vi "updateItem.vi"(0 "reference in":refnum<class "Items Controller.lvclass">, 5 "dataIN":string[](array[string]), 7 "storageIN":string[][](array[string]), 9 "IN/OUT":bool, 11 "error in (no error)":errorcluster) -> (4 "reference out":refnum<class "Items Controller.lvclass">, 6 "found?":bool, 10 "storageOUT":string[][](array[string]), 15 "error out":errorcluster)   [LabVIEW 2014, in "Items Controller.lvclass"]
uses:
  Items Controller.lvclass
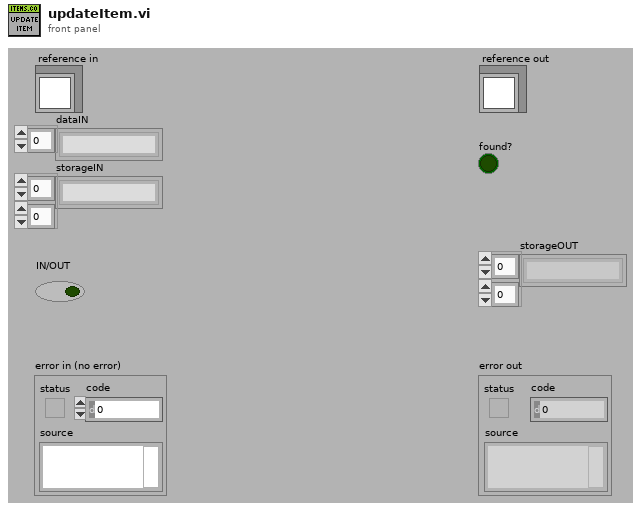
[diagram p1: front panel]
types:
  T1 = typedef "Items Controller.lvclass/ObjectAttributesRef.ctl" = refnum<data-value>
  T2 = typedef "Items Controller.lvclass/ObjectAttributes.ctl" = cluster{"MyAttribute":dbl, "data":string[][][], "file_controller_ref":refnum<class "File Controller.lvclass">, "checkIN_ref":refnum<class "checkIN.lvclass">, "checkOUT_ref":refnum<class "checkOUT.lvclass">, "item_ref":refnum<class "item.lvclass">}
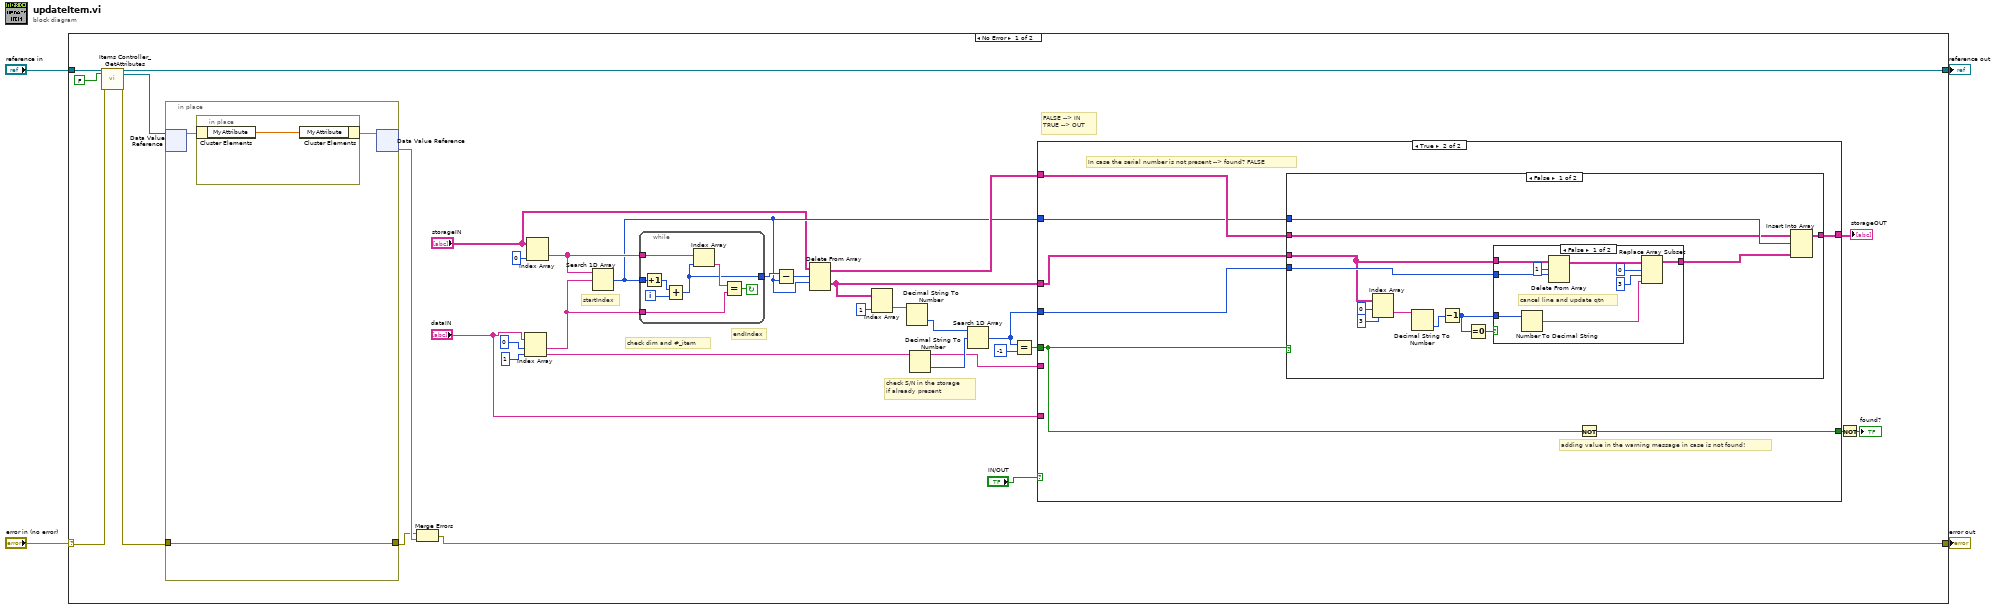
[diagram p0: block diagram]
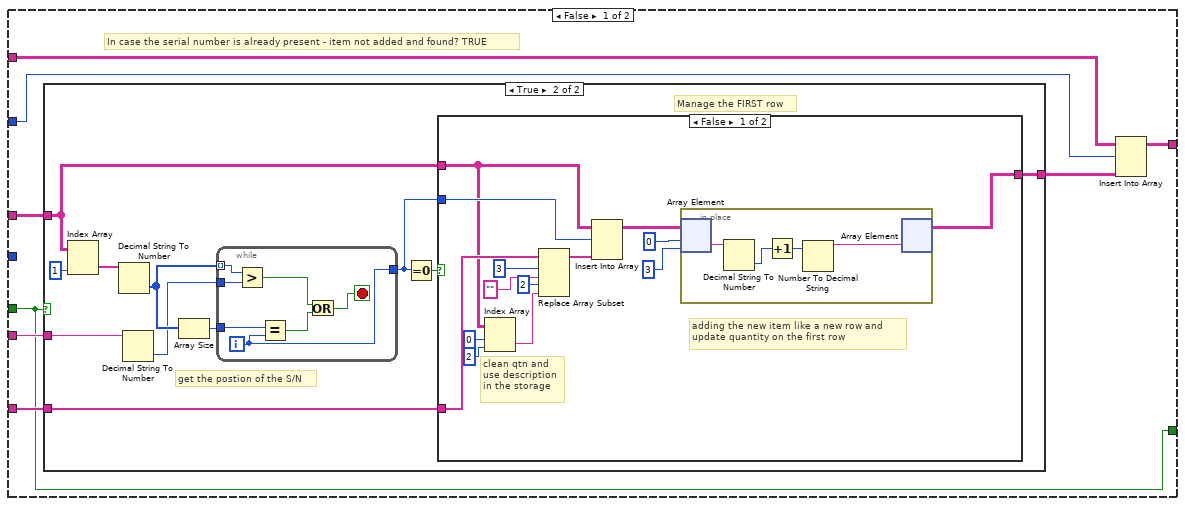
[diagram p2: hidden frame]
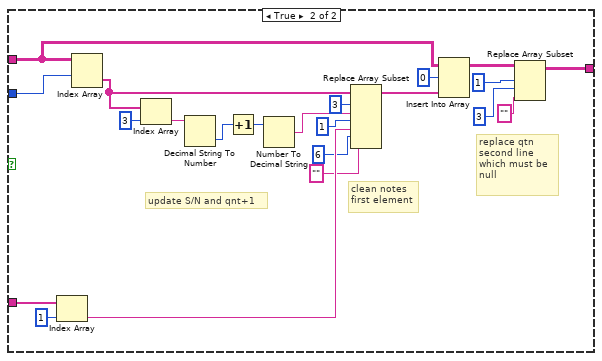
[diagram p4: hidden frame]
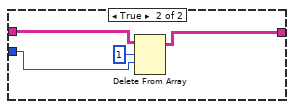
[diagram p5: hidden frame]
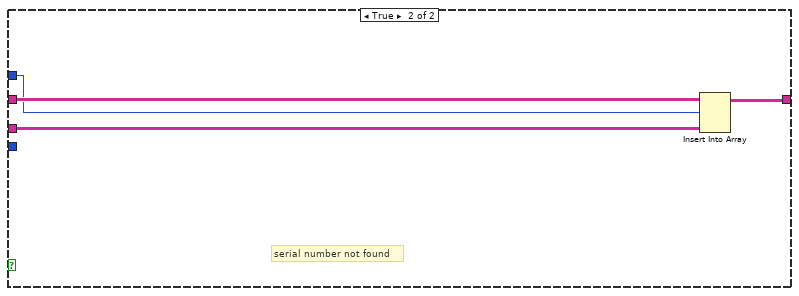
[diagram p6: hidden frame]
diagram:
  n1 = case shown="No Error" "error in (no error)" {
    selector: "error in (no error)" -> [w33 w154]
    tunnel: [w29 w154] -> w3
    tunnel: [w31 w153] -> w1
    tunnel: "reference in" -> [w35 w153]
    frame No Error {
      # "check S/N in the storage\nif already present"
      # "FALSE --> IN\nTRUE --> OUT"
      # "check dim and #_item"
      # "endIndex"
      # "startIndex"
      n2 = call "Items Controller_GetAttributes.vi"("reference in"=w35, "return data? (T)"=FALSE, "error in (no error)"=w33) -> ("reference out"=w31:refnum<class "Items Controller.lvclass">, "attributes ref"=w30:T1, "error out"=w32:errorcluster)  [unwired: 13 in, 1 out]
      n3 = in-place {
        in-place-border: w32 -> [w149]
        in-place-border: [w149] -> w36
        n4 = in-place-dvr #1(w30) -> (w150:T2)  [unwired: 1 out]
        n5 = in-place {
          n6 = in-place-cluster #2(w150) -> ("MyAttribute"=w152:dbl)
          n7 = in-place-cluster #2("MyAttribute"=w152) -> (w151:T2)
        }
        n8 = in-place-dvr #1(w151) -> (w37:errorcluster)  [unwired: 1 out]
      }
      n9 = Merge Errors(w36, w37) -> (w29:errorcluster)
      n10 = Index Array(array="dataIN", index #1=0 ("index"), index #2=1 ("index")) -> (element #1=w25:string, element #2=w13:string)
      n11 = Index Array(array="storageIN", index (col)=0 ("disabled index (col)")) -> (element=w26:string[])  [unwired: 1 in]
      n12 = Search 1D Array(1D array=w26, element=w25) -> (index of element=w20:i32)  [unwired: 1 in]
      n13 = while {
        tunnel: w26 -> [w148]
        tunnel: w20 -> [w147]
        tunnel: w25 -> [w142]
        tunnel: [w141] -> w24
        i -> [w146]
        stop <- w144 continue-if-true
        n14 = Increment(x=w147) -> (x+1=w145:i32)
        n15 = Add(x=w145, y=w146) -> (x+y=w141:i32)
        n16 = Index Array(array=w148, index=w141) -> (element=w143:string)
        n17 = Equal?(x=w143, y=w142) -> (x = y?=w144:bool)
      }
      n18 = Subtract(x=w24, y=w20) -> (x-y=w23:i32)
      n19 = Delete From Array(array="storageIN", length=w23, index (row)=w20) -> (deleted portion=w14:string[][], array with subset deleted=w21:string[][])  [unwired: 1 in]
      n20 = Index Array(array=w14, index (col)=1 ("disabled index (col)")) -> (element=w15:string[])  [unwired: 1 in]
      n21 = Decimal String To Number(string=w15) -> (number=w17:i32[])  [unwired: 2 in, 1 out]
      n22 = Decimal String To Number(string=w13) -> (number=w18:i32)  [unwired: 2 in, 1 out]
      n23 = Search 1D Array(1D array=w17, element=w18) -> (index of element=w12:i32)  [unwired: 1 in]
      n24 = Equal?(x=w12, y=-1) -> (x = y?=w11:bool)
      n25 = case shown="True" "IN/OUT" {
        tunnel: w13 -> [w45 _]
        tunnel: w14 -> [w44 w108]
        tunnel: "dataIN" -> [w43 _]
        tunnel: w21 -> [w42 w111]
        tunnel: w20 -> [w41 w110]
        tunnel: [w40 w109] -> w8
        tunnel: [w38 w105] -> w7
        tunnel: w12 -> [_ w107]
        tunnel: w11 -> [w38 w106]
        frame False {
          # "In case the serial number is already present - item not added and found? TRUE"
          n26 = case shown="True" w38 {
            tunnel: w45 -> [_ w54]
            tunnel: w44 -> [w46 w50]
            tunnel: w43 -> [_ w48]
            tunnel: [w46 w47] -> w39
            frame False {
              # "Serial number is already present"
            }
            frame True {
              # "get the postion of the S/N"
              # "Manage the FIRST row"
              n27 = Index Array(array=w50, index (col)=1 ("disabled index (col)")) -> (element=w51:string[])  [unwired: 1 in]
              n28 = Decimal String To Number(string=w51) -> (number=w55:i32[])  [unwired: 2 in, 1 out]
              n29 = Decimal String To Number(string=w54) -> (number=w53:i32)  [unwired: 2 in, 1 out]
              n30 = Array Size(array=w55) -> (size(s)=w57:i32)
              n31 = while {
                tunnel: w55 -> [w103] mode=indexing
                tunnel: w53 -> [w104]
                tunnel: [w102] -> w49
                tunnel: w57 -> [w101]
                i -> [w102]
                stop <- w99 stop-if-true
                n32 = Greater?(x=w103, y=w104) -> (0:w98:bool)
                n33 = Equal?(x=w101, y=w102) -> (x = y?=w100:bool)
                n34 = Or(x=w98, y=w100) -> (x .or. y?=w99:bool)
              }
              n35 = Equal To 0?(x=w49) -> (x = 0?=w52:bool)
              n36 = case shown="False" w52 {
                tunnel: w50 -> [w63 w85]
                tunnel: w49 -> [w71 w97]
                tunnel: w48 -> [w68 w89]
                tunnel: [w69 w78] -> w47
                frame False {
                  # "adding the new item like a new row and \nupdate quantity on the first row"
                  # "clean qtn and\nuse description\nin the storage"
                  n37 = Index Array(array=w63, index (row)=0, index (col)=2 ("disabled index (col)")) -> (element=w60:string)
                  n38 = Replace Array Subset(array=w68, new element #1="" ("new element/subarray"), index #1=3 ("index"), new element #2=w60, index #2=2 ("index")) -> (w65:string[])
                  n39 = Insert Into Array(array=w63, index (row)=w71, new element=w65) -> (w70:string[][])  [unwired: 1 in]
                  n40 = in-place {
                    n41 = in-place-array #3(w70, 0, 3) -> (w73:string)
                    n42 = Decimal String To Number(string=w73) -> (number=w75:i32)  [unwired: 2 in, 1 out]
                    n43 = Increment(x=w75) -> (x+1=w74:i32)
                    n44 = Number To Decimal String(number=w74) -> (decimal integer string=w72:string)  [unwired: 1 in]
                    n45 = in-place-array #3(w72) -> (w69:string[][])  [unwired: 2 out]
                  }
                }
                frame True {
                  # "clean notes\nfirst element"
                  # "replace qtn\nsecond line\nwhich must be\nnull"
                  # "update S/N and qnt+1"
                  n46 = Index Array(array=w89, index=1) -> (element=w86:string)
                  n47 = Index Array(array=w85, index (row)=w97) -> (element=w96:string[])  [unwired: 1 in]
                  n48 = Index Array(array=w96, index=3) -> (element=w93:string)
                  n49 = Decimal String To Number(string=w93) -> (number=w91:i32)  [unwired: 2 in, 1 out]
                  n50 = Increment(x=w91) -> (x+1=w90:i32)
                  n51 = Number To Decimal String(number=w90) -> (decimal integer string=w92:string)  [unwired: 1 in]
                  n52 = Replace Array Subset(array=w96, new element #1=w92, index #1=3 ("index"), new element #2=w86, index #2=1 ("index"), new element #3="" ("new element/subarray"), index #3=6 ("index")) -> (w83:string[])
                  n53 = Insert Into Array(array=w85, index (row)=0, new element=w83) -> (w82:string[][])  [unwired: 1 in]
                  n54 = Replace Array Subset(array=w82, new element="" ("new element/subarray"), index (row)=1, index (col)=3 ("disabled index (col)")) -> (w78:string[][])
                }
              }
            }
          }
          n55 = Insert Into Array(array=w42, index (row)=w41, new element=w39) -> (w40:string[][])  [unwired: 1 in]
        }
        frame True {
          # "adding value in the warning message in case is not found!"
          # "In case the serial number is not present --> found? FALSE"
          n56 = case shown="False" w106 {
            tunnel: w111 -> [w117 w140]
            tunnel: w107 -> [w120 _]
            tunnel: w110 -> [w119 w138]
            tunnel: [w118 w139] -> w109
            tunnel: w108 -> [w116 w137]
            frame False {
              n57 = Index Array(array=w116, index (row)=0, index (col)=3 ("disabled index (col)")) -> (element=w115:string)
              n58 = Decimal String To Number(string=w115) -> (number=w114:i32)  [unwired: 2 in, 1 out]
              n59 = Decrement(x=w114) -> (x-1=w113:i32)
              n60 = Equal To 0?(x=w113) -> (x = 0?=w112:bool)
              n61 = case shown="False" w112 {
                tunnel: [w128 w133] -> w121
                tunnel: w120 -> [w127 w136]
                tunnel: w116 -> [w126 w134]
                tunnel: w113 -> [w125 _]
                frame False {
                  # "cancel line and update qtn"
                  n62 = Number To Decimal String(number=w125) -> (decimal integer string=w124:string)  [unwired: 1 in]
                  n63 = Delete From Array(array=w126, length=1, index (row)=w127) -> (array with subset deleted=w131:string[][])  [unwired: 1 in, 1 out]
                  n64 = Replace Array Subset(array=w131, new element=w124, index (row)=0, index (col)=3 ("disabled index (col)")) -> (w128:string[][])
                }
                frame True {
                  n65 = Delete From Array(array=w134, length=1, index (row)=w136) -> (array with subset deleted=w133:string[][])  [unwired: 1 in, 1 out]
                }
              }
              n66 = Insert Into Array(array=w117, index (row)=w119, new element=w121) -> (w118:string[][])  [unwired: 1 in]
            }
            frame True {
              # "serial number not found"
              n67 = Insert Into Array(array=w140, index (row)=w138, new element=w137) -> (w139:string[][])  [unwired: 1 in]
            }
          }
          n68 = Not(x=w106) -> (.not. x?=w105:bool)
        }
      }
      "storageOUT" <- w8
      n69 = Not(x=w7) -> (.not. x?=→"found?":bool)
    }
    frame Error {
    }
  }
  "error out" <- w3
  "reference out" <- w1
